vi "Binary file create.vi"() -> ()   [LabVIEW 2015]
panel:
  out "Array":dbl[](array[numeric])
  in  "file path (use dialog)":path
  # "Binry file create"
  # "Pardeep Kumar"
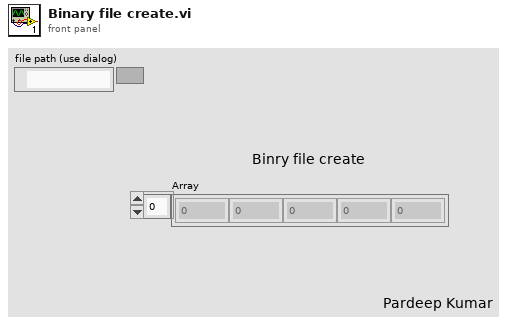
[diagram p1: front panel]
types:
  T1 = enum16{"open", "replace", "create", "open or create", "replace or create", "replace or create with confirmation"}
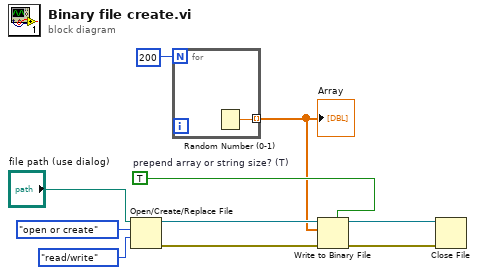
[diagram p0: block diagram]
diagram:
  w3 = TRUE  # prepend array or string size? (T)
  n1 = Open/Create/Replace File(file path (use dialog)="file path (use dialog)", operation (0:open)=T1."open or create", access (0:read/write)=enum16{"read/write", "read-only", "write-only"}."read/write") -> (refnum out=w10:refnum<file>, error out=w8:errorcluster)  [unwired: 3 in, 1 out]
  n2 = for {
    N: 200 -> [_]
    tunnel: [w11] -> w1 mode=indexing
    n3 = Random Number (0-1)() -> (number: 0 to 1=w11:dbl)
  }
  "Array" <- w1
  n4 = Write to Binary File(file (use dialog)=w10, data=w1, error in=w8, 5:w3) -> (refnum out=w9:refnum<file>, error out=w7:errorcluster)  [unwired: 2 in, 1 out]
  n5 = Close File(refnum=w9, error in=w7) -> ()  [unwired: 2 out]
